vi "Configure Marker Characteristics.vi"(5 "Marker Trace (1: Trace 1)":u16(ring)=1 items=["Trace 1"=1, "Trace 2"=2, "Trace 3"=3], 7 "Function (1: Band Power)":u16(ring)=1 items=["Off", "Band Power", "Marker Noise"], 8 "error in (no error)":errorcluster, 9 "Enable Continuous Peaking (T: Enable)":bool=TRUE, 10 "Active Marker (1: Marker1)":u16(ring)=1 items=["Marker1"=1, "Marker2"=2, "Marker3"=3, "Marker4"=4], 11 "VISA resource name":refnum<visa-resource-name>) -> (0 "error out":errorcluster, 3 "VISA resource name out":refnum<visa-resource-name>)   [LabVIEW 2014, in "Agilent ESA PSA Series.lvlib"]
doc: "Configures the marker settings."
uses:
  Agilent ESA PSA Series.lvlib
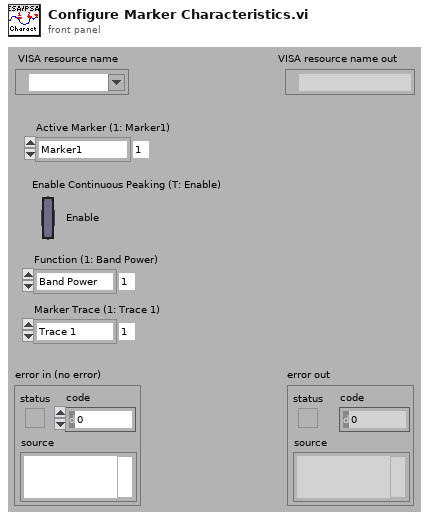
[diagram p1: front panel]
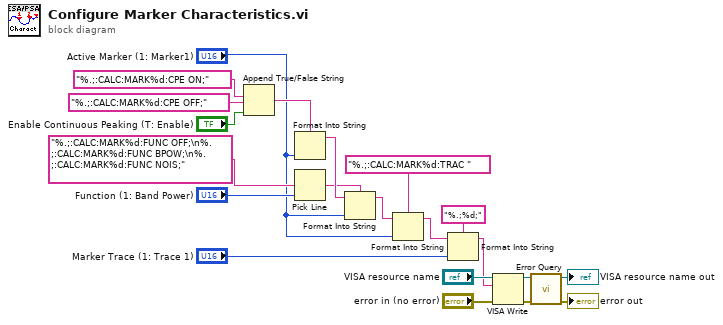
[diagram p0: block diagram]
diagram:
  n1 = Append True/False String(1:"Enable Continuous Peaking (T: Enable)", 2:"%.;:CALC:MARK%d:CPE OFF;" ("false string"), 3:"%.;:CALC:MARK%d:CPE ON;" ("false string")) -> (0:w12:string)  [unwired: 1 in]
  n2 = Format Into String(format string=w12, "Active Marker (1: Marker1)") -> (resulting string=w9:string)  [unwired: 2 in, 1 out]
  n3 = Pick Line(multi-line string="%.;:CALC:MARK%d:FUNC OFF;\n%.;:CALC:MARK%d:FUNC BPOW;\n%.;:CALC:MARK%d:FUNC NOIS;" ("false string"), line index="Function (1: Band Power)") -> (output string=w8:string)  [unwired: 1 in]
  n4 = Format Into String(format string=w8, initial string=w9, "Active Marker (1: Marker1)") -> (resulting string=w3:string)  [unwired: 1 in, 1 out]
  n5 = Format Into String(format string="%.;:CALC:MARK%d:TRAC ", initial string=w3, "Active Marker (1: Marker1)") -> (resulting string=w5:string)  [unwired: 1 in, 1 out]
  n6 = Format Into String(format string="%.;%d;", initial string=w5, "Marker Trace (1: Trace 1)") -> (resulting string=w2:string)  [unwired: 1 in, 1 out]
  n7 = VISA Write(VISA resource name="VISA resource name", write buffer=w2, error in (no error)="error in (no error)") -> (VISA resource name out=w19:refnum<visa-resource-name>, error out=w17:errorcluster)  [unwired: 1 out]
  n8 = call "Error Query.vi"("error in (no error)"=w17, "VISA resource name"=w19) -> ("error out"=→"error out":errorcluster, "VISA resource name out"=→"VISA resource name out":refnum<visa-resource-name>)  [unwired: 6 in, 2 out]
